vi "HXG2_Alarm Parser.vi"(7 "Clear Alarms Ref":refnum<vi>, 8 "error in (no error)":errorcluster, 9 "Alarm Cluster In":T1, 10 "Analog In":T3, 11 "Digital In":T4) -> (0 "error out":errorcluster, 3 "Alarm Cluster":T1)   [LabVIEW 2012]
doc: "This VI processes all hardware information to display Alarms. It uses two FGV timers for the blower and the pump to decide if there is a drive fault."
uses:
  Controls/HXG2_DigitalIn.ctl
  Controls/HXG2_AnalogIn.ctl
  Controls/HXG2_AlarmCluster.ctl
  Controls/UI/HXG2_LED.ctl
  Modules/EnableAirGly/HXG2enable.ctl
  Modules/Timers/HXG2_BlowerPumpl.ctl
  Modules/CompressorContactor/HXG2comp.ctl
panel:
  out "Clear Alarms 2":bool
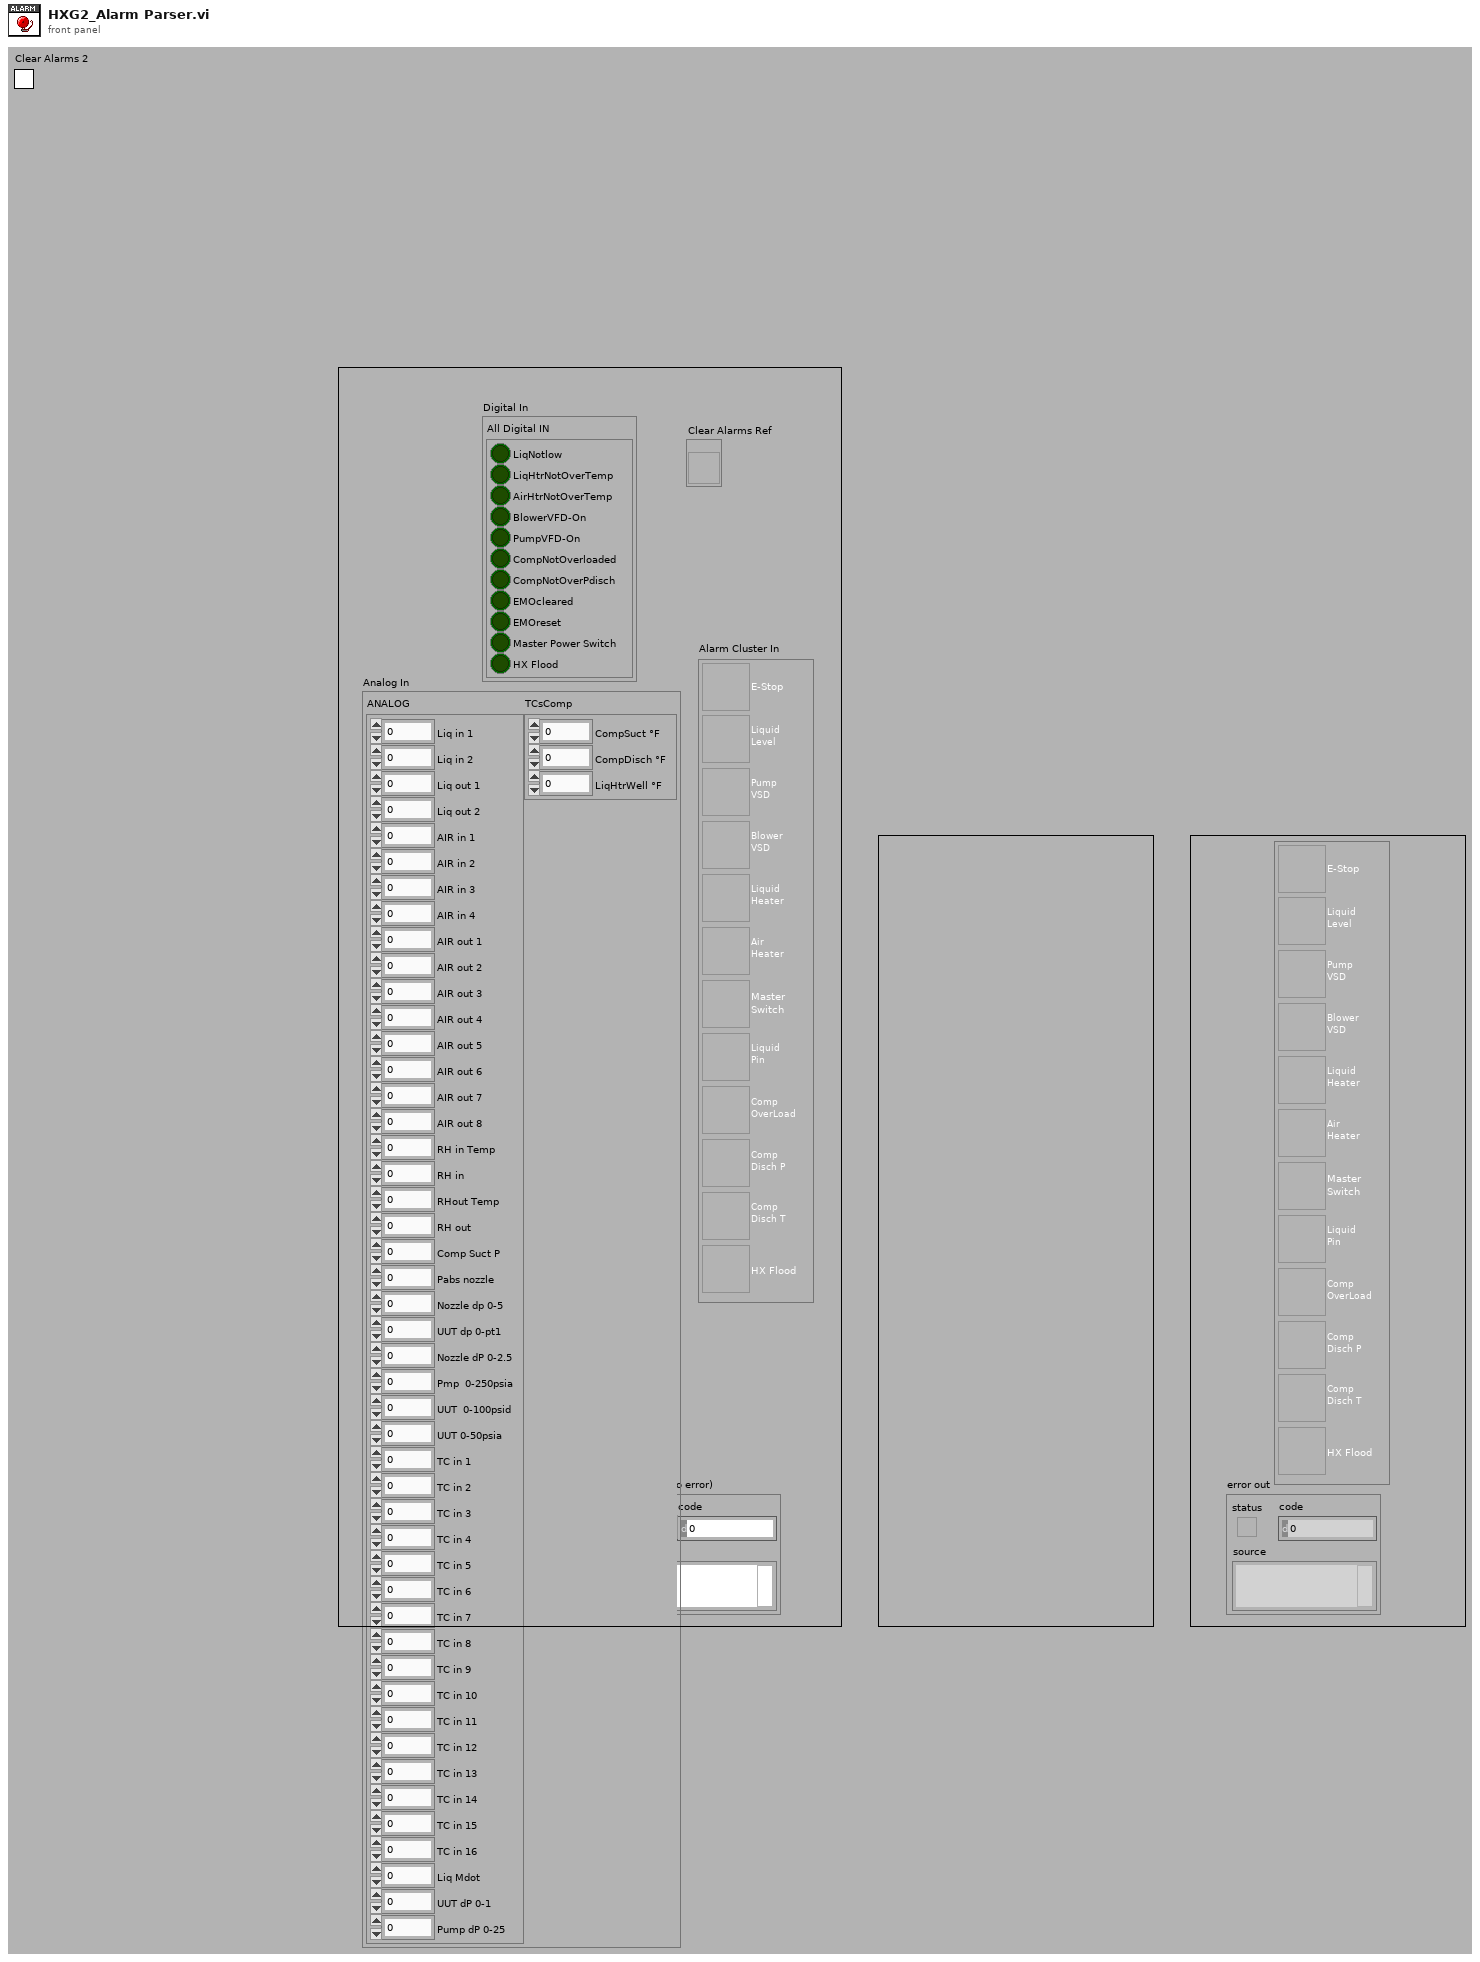
[diagram p1: front panel]
types:
  T1 = typedef "HXG2_AlarmCluster.ctl" = cluster{"E-Stop":T2, "Liquid\nLevel":T2, "Pump\nVSD":T2, "Blower\nVSD":T2, "Liquid\nHeater":T2, "Air\nHeater":T2, "Master\nSwitch":T2, "Liquid\nPin":T2, "Comp\nOverLoad":T2, "Comp\nDisch P":T2, "Comp \nDisch T":T2, "HX Flood":T2}
  T2 = typedef "HXG2_LED.ctl" = bool
  T3 = typedef "HXG2_AnalogIn.ctl" = cluster{"ANALOG":cluster{"Liq in 1":dbl, "Liq in 2":dbl, "Liq out 1":dbl, "Liq out 2":dbl, "AIR in 1":dbl, "AIR in 2":dbl, "AIR in 3":dbl, "AIR in 4":dbl, "AIR out 1":dbl, "AIR out 2":dbl, "AIR out 3":dbl, "AIR out 4":dbl, "AIR out 5":dbl, "AIR out 6":dbl, "AIR out 7":dbl, "AIR out 8":dbl, "RH in Temp":dbl, "RH in":dbl, "RHout Temp":dbl, "RH out":dbl, "Comp Suct P":dbl, "Pabs nozzle":dbl, "Nozzle dp 0-5":dbl, "UUT dp 0-pt1":dbl, "Nozzle dP 0-2.5":dbl, "Pmp  0-250psia":dbl, "UUT  0-100psid":dbl, "UUT 0-50psia":dbl, "TC in 1":dbl, "TC in 2":dbl, "TC in 3":dbl, "TC in 4":dbl, "TC in 5":dbl, "TC in 6":dbl, "TC in 7":dbl, "TC in 8":dbl, "TC in 9":dbl, "TC in 10":dbl, "TC in 11":dbl, "TC in 12":dbl, "TC in 13":dbl, "TC in 14":dbl, "TC in 15":dbl, "TC in 16":dbl, "Liq Mdot":dbl, "UUT dP 0-1":dbl, "Pump dP 0-25":dbl}, "TCsComp":cluster{"CompSuct °F  ":dbl, "CompDisch °F":dbl, "LiqHtrWell °F":dbl}}
  T4 = typedef "HXG2_DigitalIn.ctl" = cluster{"All Digital IN":cluster{"LiqNotlow":bool, "LiqHtrNotOverTemp":bool, "AirHtrNotOverTemp":bool, "BlowerVFD-On":bool, "PumpVFD-On":bool, "CompNotOverloaded":bool, "CompNotOverPdisch":bool, "EMOcleared":bool, "EMOreset":bool, "Master Power Switch":bool, "HX Flood":bool}}
  T5 = typedef "HXG2enable.ctl" = enum16{"Write Refs", "Write", "Pass"}
  T6 = typedef "HXG2_BlowerPumpl.ctl" = enum16{"Stop", "Start", "Check Time"}
  T7 = cluster{"Air-Liq Out[0]":bool, "Air-Liq Out[1]":bool, "Air-Liq Out[2]":bool, "Air-Liq Out[3]":bool, "Air-Liq Out[4]":bool, "Air-Liq Out[5]":bool, "Air-Liq Out[6]":bool, "Air-Liq Out[7]":bool, "Air-Liq Out[8]":bool}
  T8 = typedef "HXG2comp.ctl" = enum16{"Write", "Pass"}
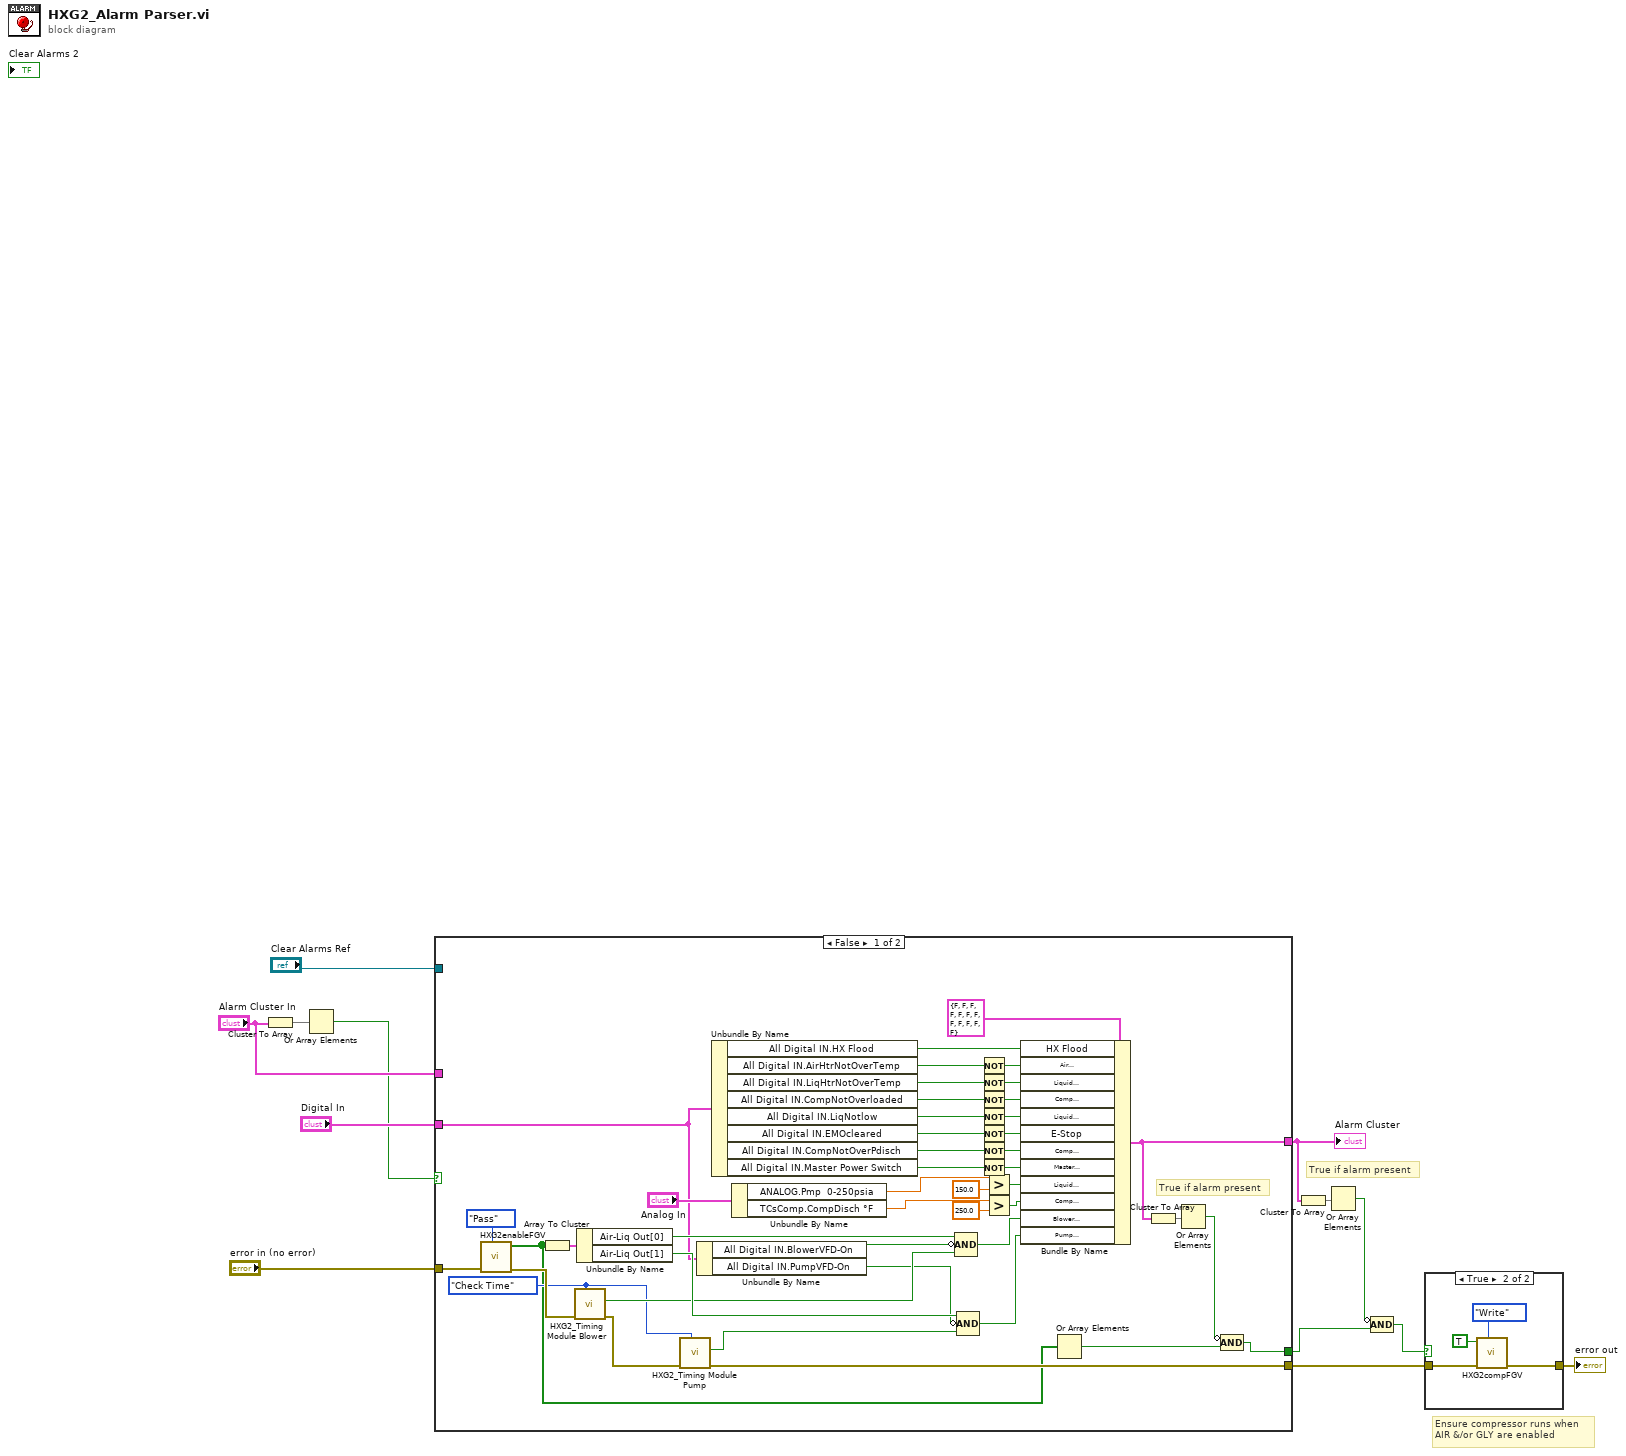
[diagram p0: block diagram]
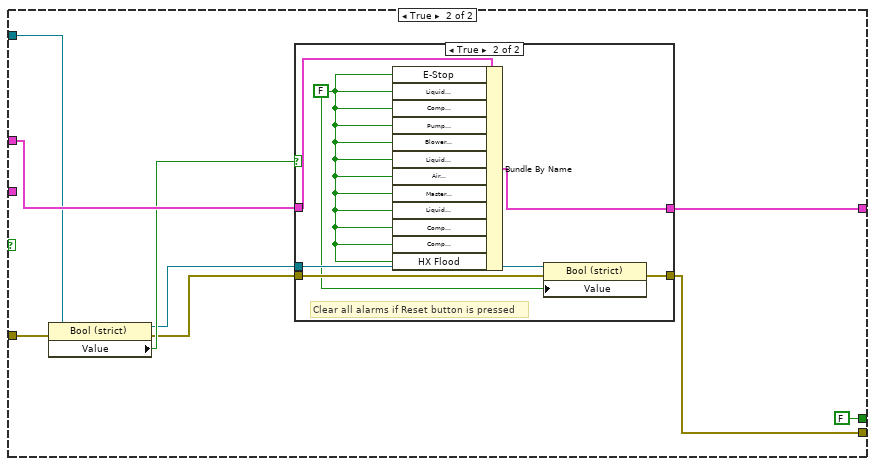
[diagram p2: hidden frame]
diagram:
  # "True if alarm present"
  # "Ensure compressor runs when\nAIR &/or GLY are enabled"
  n1 = Cluster To Array(cluster="Alarm Cluster In") -> (array=w10:T2[])
  n2 = Or Array Elements(Boolean array=w10) -> (logical OR=w3:bool)
  n3 = case shown="False" w3 {
    tunnel: "Digital In" -> [w32 _]
    tunnel: "error in (no error)" -> [w22 w64]
    tunnel: [w20 w59] -> w12
    tunnel: [w16 FALSE] -> w5
    tunnel: [w14 w65] -> w4
    tunnel: "Alarm Cluster In" -> [_ w66]
    tunnel: "Clear Alarms Ref" -> [_ w63]
    frame False {
      w23 = HXG2_BlowerPumpl."Check Time" ("Timer Command")
      # "True if alarm present"
      n4 = call "HXG2enableFGV.vi"("ENABLE Ctrl"=HXG2enable."Pass" ("ENABLE"), "error in (no error)"=w22) -> ("error out"=w31:errorcluster, "Air-Liq Out"=w19:bool[])  [unwired: 7 in, 1 out]
      n5 = Array To Cluster(array=w19) -> (cluster=w35:T7)
      n6 = call "HXG2_Timing Module Blower.vi"("Timer Command"=w23, "error in (no error)"=w31) -> ("error out"=w30:errorcluster, "Done?"=w28:bool)  [unwired: 7 in, 1 out]
      n7 = Unbundle By Name(w35) -> ("Air-Liq Out[0]"=w34:bool, "Air-Liq Out[1]"=w33:bool)
      n8 = call "HXG2_Timing Module Pump.vi"("Timer Command"=w23, "error in (no error)"=w30) -> ("error out"=w20:errorcluster, "Done?"=w26:bool)  [unwired: 7 in, 1 out]
      n9 = Unbundle By Name(w32) -> ("All Digital IN.BlowerVFD-On"=w29:bool, "All Digital IN.PumpVFD-On"=w25:bool)
      n10 = Unbundle By Name(w32) -> ("All Digital IN.HX Flood"=w15:bool, "All Digital IN.AirHtrNotOverTemp"=w56:bool, "All Digital IN.LiqHtrNotOverTemp"=w54:bool, "All Digital IN.CompNotOverloaded"=w52:bool, "All Digital IN.LiqNotlow"=w50:bool, "All Digital IN.EMOcleared"=w48:bool, "All Digital IN.CompNotOverPdisch"=w46:bool, "All Digital IN.Master Power Switch"=w44:bool)
      n11 = Unbundle By Name("Analog In") -> ("ANALOG.Pmp  0-250psia"=w40:dbl, "TCsComp.CompDisch °F"=w39:dbl)
      n12 = Compound Arithmetic op=AND(w34, invert w29, w28) -> (w27:bool)
      n13 = Compound Arithmetic op=AND(w33, invert w25, w26) -> (w24:bool)
      n14 = Not(x=w56) -> (.not. x?=w55:bool)
      n15 = Not(x=w54) -> (.not. x?=w53:bool)
      n16 = Not(x=w52) -> (.not. x?=w51:bool)
      n17 = Not(x=w50) -> (.not. x?=w49:bool)
      n18 = Not(x=w48) -> (.not. x?=w47:bool)
      n19 = Not(x=w46) -> (.not. x?=w45:bool)
      n20 = Not(x=w44) -> (.not. x?=w43:bool)
      n21 = Greater?(x=w40, y=150.0) -> (0:w38:bool)
      n22 = Greater?(x=w39, y=250.0) -> (0:w37:bool)
      n23 = Bundle By Name(cluster=T1 {"E-Stop"=FALSE, "Liquid\nLevel"=FALSE, "Pump\nVSD"=FALSE, "Blower\nVSD"=FALSE, "Liquid\nHeater"=FALSE, "Air\nHeater"=FALSE, "Master\nSwitch"=FALSE, "Liquid\nPin"=FALSE, "Comp\nOverLoad"=FALSE, "Comp\nDisch P"=FALSE, "Comp \nDisch T"=FALSE, "HX Flood"=FALSE} ("Alarm Cluster"), "HX Flood"=w15, "Air\nHeater"=w55, "Liquid\nHeater"=w53, "Comp\nOverLoad"=w51, "Liquid\nLevel"=w49, "E-Stop"=w47, "Comp\nDisch P"=w45, "Master\nSwitch"=w43, "Liquid\nPin"=w38, "Comp \nDisch T"=w37, "Blower\nVSD"=w27, "Pump\nVSD"=w24) -> (w14:T1)
      n24 = Or Array Elements(Boolean array=w19) -> (logical OR=w17:bool)
      n25 = Cluster To Array(cluster=w14) -> (array=w21:T2[])
      n26 = Or Array Elements(Boolean array=w21) -> (logical OR=w18:bool)
      n27 = Compound Arithmetic op=AND(invert w18, w17) -> (w16:bool)
    }
    frame True {
      n28 = property class="Bool (strict)"(reference=w63, error in=w64) -> (reference out=w60:refnum<vi>, error out=w61:errorcluster, "Value"=w62:bool)
      n29 = case shown="True" w62 {
        tunnel: w66 -> [w69 w75]
        tunnel: [w69 w74] -> w65
        tunnel: w61 -> [w68 w73]
        tunnel: w60 -> [_ w72]
        tunnel: [w68 w71] -> w59
        frame False {
        }
        frame True {
          w70 = FALSE
          # "Clear all alarms if Reset button is pressed"
          n30 = Bundle By Name(cluster=w75, "E-Stop"=w70, "Liquid\nLevel"=w70, "Comp\nOverLoad"=w70, "Pump\nVSD"=w70, "Blower\nVSD"=w70, "Liquid\nHeater"=w70, "Air\nHeater"=w70, "Master\nSwitch"=w70, "Liquid\nPin"=w70, "Comp \nDisch T"=w70, "Comp\nDisch P"=w70, "HX Flood"=w70) -> (w74:T1)
          n31 = property class="Bool (strict)"(reference=w72, error in=w73, "Value"=w70) -> (error out=w71:errorcluster)  [unwired: 1 out]
        }
      }
    }
  }
  "Alarm Cluster" <- w4
  n32 = Cluster To Array(cluster=w4) -> (array=w7:T2[])
  n33 = Or Array Elements(Boolean array=w7) -> (logical OR=w8:bool)
  n34 = Compound Arithmetic op=AND(invert w8, w5) -> (w6:bool)
  n35 = case shown="True" w6 {
    tunnel: w12 -> [w76 w80]
    tunnel: [w76 w79] -> w11
    frame False {
    }
    frame True {
      n36 = call "HXG2compFGV.vi"("CompFGV"=HXG2comp."Write", "error in (no error)"=w80, "RUN?"=TRUE) -> ("error out"=w79:errorcluster)  [unwired: 7 in, 1 out]
    }
  }
  "error out" <- w11
